vi "move_zip.vi"(6 "zip_move_directory":path, 8 "error in (no error)":errorcluster, 11 "build_specifications":T1={"type"=enum."zip", "build_spec_name"="em-lv-NetworkStreams_Static", "target_name"="My Computer", "owner_name []"=[], "project_path"=path "D:/SourceControl/vi-packages/EM NetworkStreams/Source/NetworkStreams_Static/em-lv-NetworkStreams_Static.lvproj", "build_destination"=path "D:/SourceControl/vi-packages/EM NetworkStreams/Distribution/2014", "build_artifact"=path ""}) -> (0 "error out":errorcluster)   [LabVIEW 2015, in "lv-builder-default.lvlib"]
uses:
  lv-builder-default.lvlib
  lv-build/public/_controls/build_specification.ctl
  lv-build/public/_controls/build_type.ctl
  <userlib>/antonio-alexander/lv-bin/public/api/v1/v1.lvlib
  lv-build/lv-build.lvlib
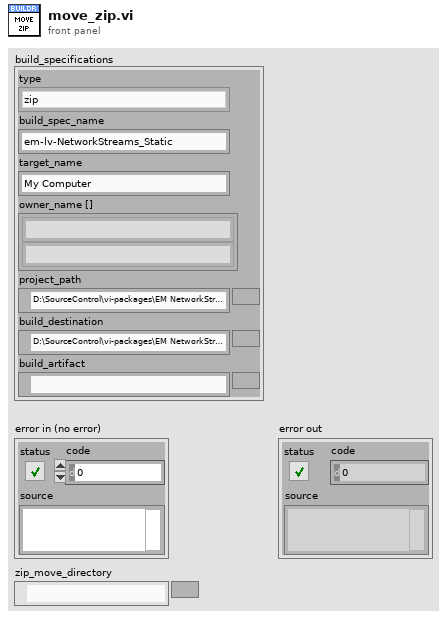
[diagram p1: front panel]
types:
  T1 = typedef "lv-build.lvlib/build_specification.ctl" = cluster{"type":T2, "build_spec_name":string, "target_name":string, "owner_name []":string[], "project_path":path, "build_destination":path, "build_artifact":path}
  T2 = typedef "lv-build.lvlib/build_type.ctl" = enum16{"<build_type>", "application_pc", "application_rt", "installer", "llb", "lvlibp", "zip", "fpga", "<null>"}
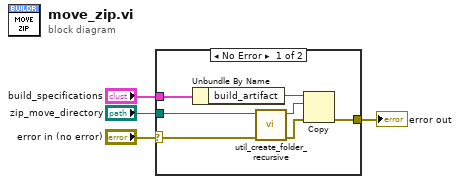
[diagram p0: block diagram]
diagram:
  n1 = case shown="No Error" "error in (no error)" {
    selector: "error in (no error)" -> [w7 w12]
    tunnel: "build_specifications" -> [w11 _]
    tunnel: [w5 w12] -> w3
    tunnel: "zip_move_directory" -> [w10 _]
    frame No Error {
      n2 = Unbundle By Name(w11) -> ("build_artifact"=w9:path)
      n3 = call <userlib>:"util_create_folder_recursive.vi"("error in"=w7, "path in"=w10) -> ("error out"=w6:errorcluster, "path out"=w8:path)  [unwired: 8 in]
      n4 = Copy(8:w6, 10:w8, 11:w9) -> (0:w5:errorcluster)  [unwired: 2 in, 2 out]
    }
    frame Error {
    }
  }
  "error out" <- w3
